vi "File.Rotate.Scheduler.vi"(8 "error in (no error)":errorcluster, 11 "File.Rotate in":refnum<class "File.Rotate.lvclass">) -> (0 "error out":errorcluster, 3 "File.Rotate out":refnum<class "File.Rotate.lvclass">)   [LabVIEW 2024, in "EQMF.lvlib" / "File Utils.lvlib" / "File.Rotate.lvclass"]
uses:
  File.Rotate.lvclass
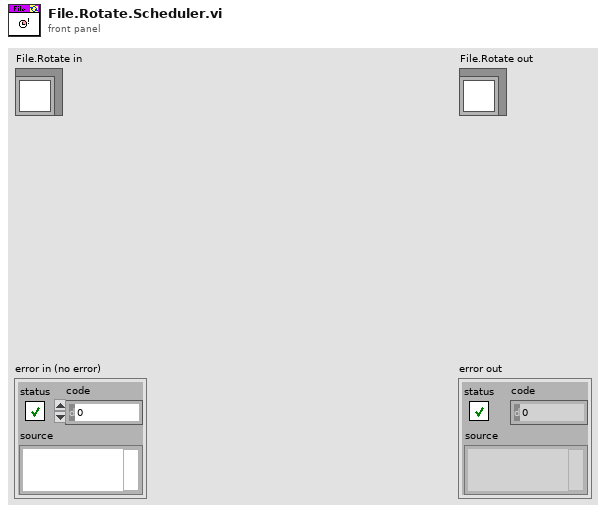
[diagram p1: front panel]
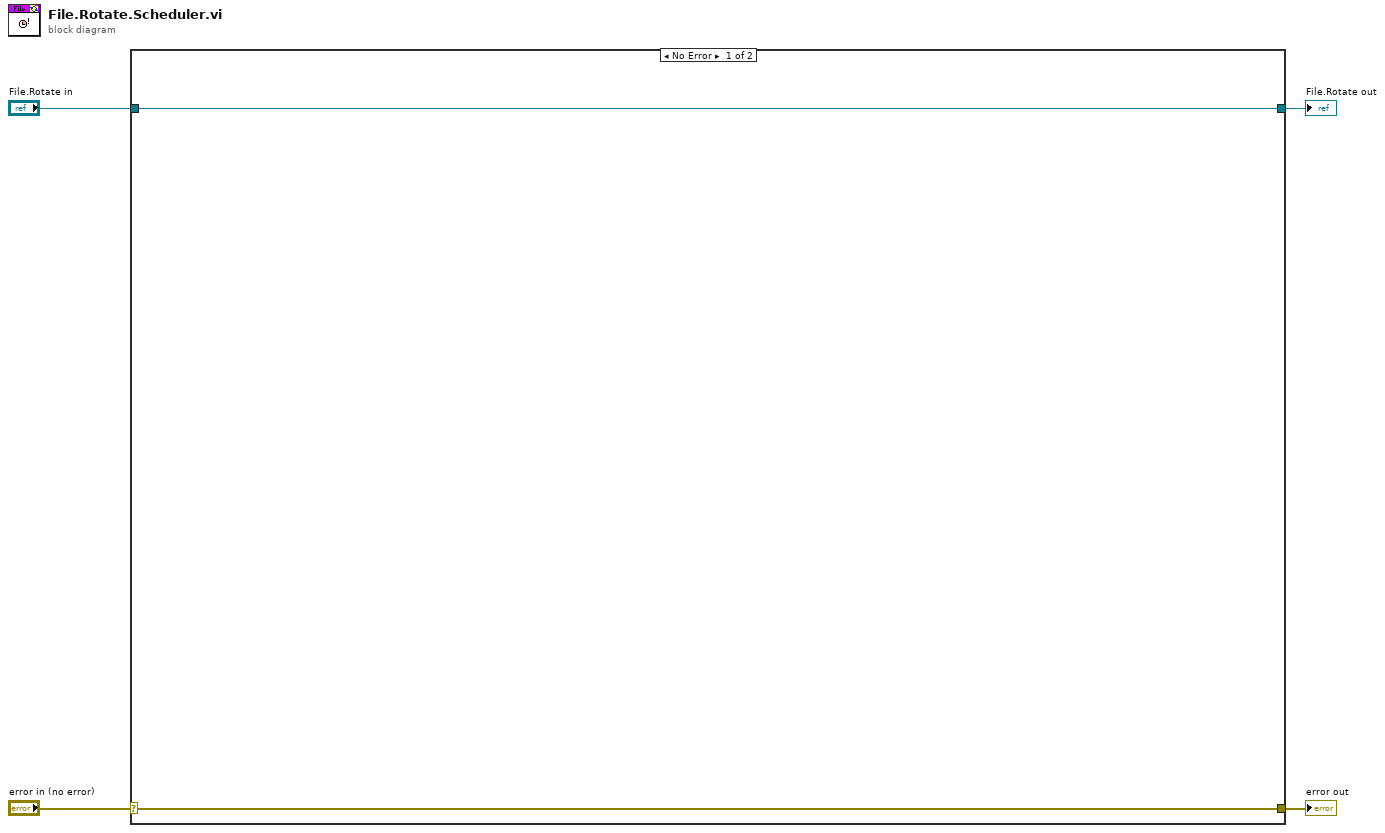
[diagram p0: block diagram]
diagram:
  n1 = case shown="No Error" "error in (no error)" {
    selector: "error in (no error)" -> [w5 w8]
    tunnel: [w5 w8] -> w3
    tunnel: [w6 w7] -> w1
    tunnel: "File.Rotate in" -> [w6 w7]
    frame No Error {
    }
    frame Error {
    }
  }
  "error out" <- w3
  "File.Rotate out" <- w1
